vi "Test SUBACK packet.vi"() -> ()   [LabVIEW 2013]
uses:
  source/Control Packets/SUBACK/SUBACK.lvclass
  source/Control Packets/SUBACK/Subscription Success Code.ctl
  source/Control Packets/ControlPacket/QualityOfService -- enum.ctl
  source/Control Packets/ControlPacket/ControlPacket.lvclass/ControlPacket.ctl
  source/Control Packets/ControlPacket/ControlPacket.lvclass
panel:
  out "Return Codes":bool
  out "Packet ID":u16 format="%04x"
  out "error out":errorcluster
  out "Packet Identifier":bool
  out "Packet type":bool
  out "All packets consumed":bool
  out "Complete Packet":bool
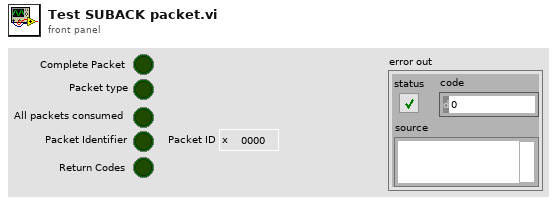
[diagram p1: front panel]
types:
  T1 = typedef "SUBACK.lvclass/Subscription Success Code.ctl" = cluster{"Subscription Failure":bool, "QoS":T2}
  T2 = typedef "ControlPacket.lvclass/QualityOfService -- enum.ctl" = enum16{"0 (At Most Once)", "1 (At Least Once)", "2 (Exactly Once)"}
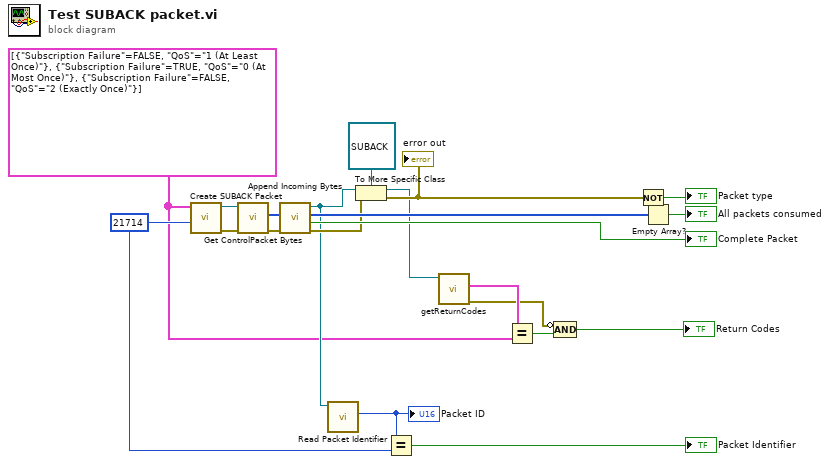
[diagram p0: block diagram]
diagram:
  w4 = T1[] [{"Subscription Failure"=FALSE, "QoS"=enum."1 (At Least Once)"}, {"Subscription Failure"=TRUE, "QoS"=enum."0 (At Most Once)"}, {"Subscription Failure"=FALSE, "QoS"=enum."2 (Exactly Once)"}] ("Return Codes")
  w9 = u16 21714 ("Packet ID")
  n1 = call "Create SUBACK Packet.vi"("Packet ID"=w9, "Return Codes"=w4) -> ("error out"=w8:errorcluster, "SUBACK"=w7:refnum<class "SUBACK.lvclass">)  [unwired: 8 in]
  n2 = call "Get ControlPacket Bytes.vi"("error in (no error)"=w8, "ControlPacket"=w7) -> ("error out"=w15:errorcluster, "Bytes Stream"=w21:u8[])  [unwired: 7 in, 1 out]
  n3 = call "Append Incoming Bytes.vi"("error in (no error)"=w15, "Incoming Packets"=w21) -> ("error out"=w14:errorcluster, "Complete Packet"=→"Complete Packet":bool, "Remaining Packets"=w19:u8[], "ControlPacket"=w11:refnum<class "ControlPacket.lvclass">)  [unwired: 6 in]
  n4 = call "Read Packet Identifier.vi"("ControlPacket in"=w11) -> ("Packet Identifier"=w13:u16)  [unwired: 9 in, 1 out]
  "Packet ID" <- w13
  n5 = To More Specific Class(target class=refnum<class "SUBACK.lvclass"> refnum ("SUBACK.lvclass"), reference=w11, error in=w14) -> (specific class reference=w6:refnum<class "SUBACK.lvclass">, error out=w17:errorcluster)
  "error out" <- w17
  n6 = Equal?(x=w13, y=w9) -> (x = y?=→"Packet Identifier":bool)
  n7 = call "getReturnCodes.vi"("SUBACK in"=w6) -> ("error out"=w2:errorcluster, "Subscription Success"=w5:T1[])  [unwired: 8 in, 1 out]
  n8 = Equal?(x=w5, y=w4) -> (x = y?=w3:bool)
  n9 = Compound Arithmetic op=AND(invert w2, w3) -> (→"Return Codes":bool)
  n10 = Not(x=w17) -> (.not. x?=→"Packet type":bool)
  n11 = Empty Array?(array=w19) -> (empty?=→"All packets consumed":bool)
